vi "Merge Config.vi"(5 "Overwrite excisting? [F]":bool, 6 "Carya Config source in":refnum<class "Carya Config.lvclass">, 7 "Section name/Regex":string, 8 "error in (no error)":errorcluster, 10 "Use Section Regex? [T]":bool=TRUE, 11 "Carya Config dest in":refnum<class "Carya Config.lvclass">) -> (0 "error out":errorcluster, 3 "Carya Config dest out":refnum<class "Carya Config.lvclass">, 4 "Carya Config source out":refnum<class "Carya Config.lvclass">)   [LabVIEW 2013, in "Carya Config.lvclass"]
doc: "Copyright 2018, Carya Automatisering, Wiebe Walstra."
uses:
  Carya Config.lvclass
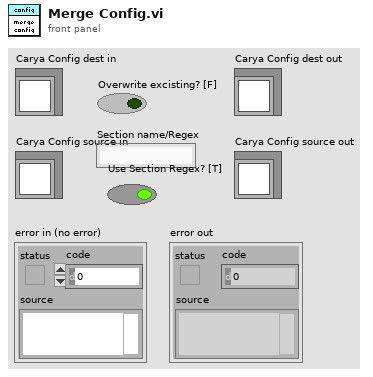
[diagram p1: front panel]
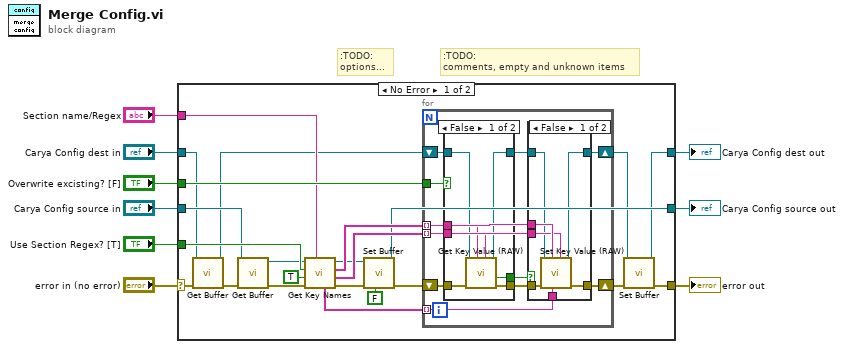
[diagram p0: block diagram]
diagram:
  # ":TODO:\ncomments, empty and unknown items"
  # ":TODO:\noptions..."
  n1 = case shown="No Error" "error in (no error)" {
    selector: "error in (no error)" -> [w22 w64]
    tunnel: [w26 w64] -> w8
    tunnel: [w24 w63] -> w6
    tunnel: "Carya Config dest in" -> [w19 w63]
    tunnel: "Carya Config source in" -> [w20 w62]
    tunnel: [w25 w62] -> w4
    tunnel: "Overwrite excisting? [F]" -> [w29 _]
    tunnel: "Section name/Regex" -> [w28 _]
    tunnel: "Use Section Regex? [T]" -> [w27 _]
    frame No Error {
      n2 = call-dynamic "Get Buffer.vi"("error in (no error)"=w22, "Carya Config in"=w19) -> ("error out"=w23:errorcluster, "Config"=w18:refnum<class "Carya Config.lvclass">)  [unwired: 8 in]
      n3 = call-dynamic "Get Buffer.vi"("error in (no error)"=w23, "Carya Config in"=w20) -> ("error out"=w21:errorcluster, "Config"=w16:refnum<class "Carya Config.lvclass">)  [unwired: 8 in]
      n4 = call-dynamic "Get Key Names.vi"("Section name/Regex"=w28, "error in (no error)"=w21, "Use Key Regex? [F]"=TRUE ("Use Section Regex? [F]"), "Use Section Regex? [F]"=w27, "Carya Config in"=w16) -> ("error out"=w12:errorcluster, "Key names"=w30:string[], "Section names"=w31:string[], "Carya Config out"=w14:refnum<class "Carya Config.lvclass">, "Context (concatenated)"=w15:string[])  [unwired: 2 in]
      n5 = call-dynamic "Set Buffer.vi"("Set? [T]"=FALSE, "error in (no error)"=w12, "Carya Config"=w14) -> ("error out"=w11:errorcluster, "Carya Config out"=w25:refnum<class "Carya Config.lvclass">)  [unwired: 7 in]
      n6 = for {
        tunnel: w31 -> [w33] mode=indexing
        tunnel: w30 -> [w40] mode=indexing
        shift-right: [w42] -> w17
        shift-left: w18 -> [w43]
        shift-right: [w41] -> w13
        shift-left: w11 -> [w34]
        tunnel: w29 -> [w39]
        tunnel: w15 -> [w36] mode=indexing
        n7 = case shown="False" w39 {
          tunnel: w43 -> [w50 w52]
          tunnel: [w49 w52] -> w38
          tunnel: w33 -> [w48 _]
          tunnel: w40 -> [w47 _]
          tunnel: [w46 _] -> w37
          tunnel: [w45 w51] -> w35
          tunnel: w34 -> [w44 w51]
          frame False {
            n8 = call-dynamic "Get Key Value (RAW).vi"("Key name"=w47, "Section name"=w48, "error in (no error)"=w44, "Carya Config in"=w50) -> ("error out"=w45:errorcluster, "Found?"=w46:bool, "Carya Config out"=w49:refnum<class "Carya Config.lvclass">)  [unwired: 4 in, 1 out]
          }
          frame True {
          }
        }
        n9 = case shown="False" w37 {
          tunnel: [w59 w61] -> w42
          tunnel: [w58 w60] -> w41
          tunnel: w33 -> [w57 _]
          tunnel: w40 -> [w56 _]
          tunnel: w38 -> [w55 w61]
          tunnel: w36 -> [w54 _]
          tunnel: w35 -> [w53 w60]
          frame False {
            n10 = call-dynamic "Set Key Value (RAW).vi"("Key name"=w56, "Key value"=w54, "Section name"=w57, "error in (no error)"=w53, "Carya Config in"=w55) -> ("error out"=w58:errorcluster, "Carya Config out"=w59:refnum<class "Carya Config.lvclass">)  [unwired: 2 in, 3 out]
          }
          frame True {
          }
        }
      }
      n11 = call-dynamic "Set Buffer.vi"("error in (no error)"=w13, "Carya Config"=w17) -> ("error out"=w26:errorcluster, "Carya Config out"=w24:refnum<class "Carya Config.lvclass">)  [unwired: 8 in]
    }
    frame Error {
    }
  }
  "error out" <- w8
  "Carya Config dest out" <- w6
  "Carya Config source out" <- w4
